vi "Cal Attendance.vi"(8 "error in (no error)":errorcluster, 11 "AttendRecord.lvclass":refnum<class "AttendRecord.lvclass">) -> (0 "error out":errorcluster, 3 "AttendRecord.lvclass":refnum<class "AttendRecord.lvclass">)   [LabVIEW 2015]
uses:
  AttendRecord.lvclass
panel:
  in  "Calendances(\"\")":string[][](array[string])
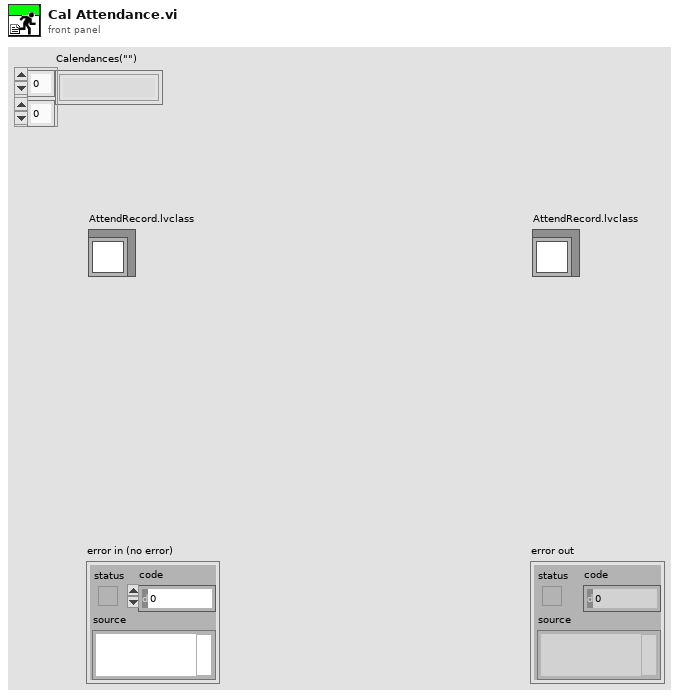
[diagram p1: front panel]
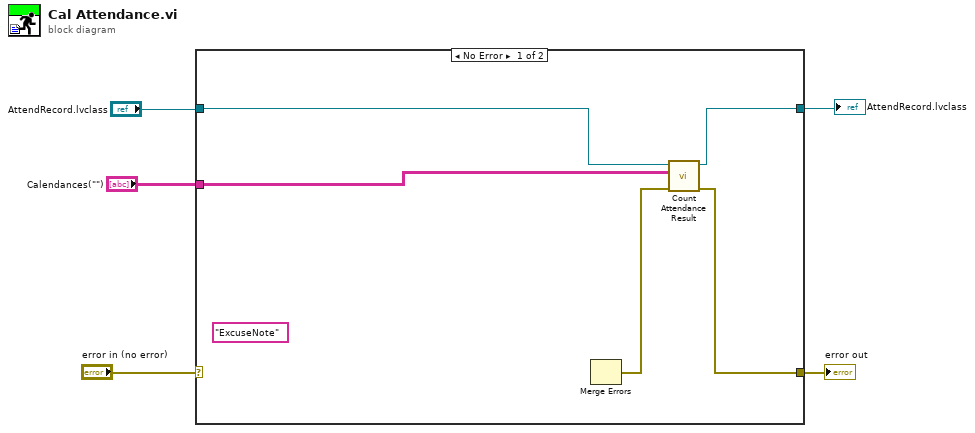
[diagram p0: block diagram]
diagram:
  n1 = case shown="No Error" "error in (no error)" {
    selector: "error in (no error)" -> [_ w12]
    tunnel: [w9 w12] -> w4
    tunnel: [w7 w11] -> w2
    tunnel: "AttendRecord.lvclass" -> [w8 w11]
    tunnel: "Calendances(\"\")" -> [w6 _]
    frame No Error {
      (unwired) "ExcuseNote" ("string")
      n2 = Merge Errors() -> (w10:errorcluster)  [unwired: 3 in]
      n3 = call "Count Attendance Result.vi"("error in (no error)"=w10, "Calendances(\"\")"=w6, "AttendRecord.lvclass"=w8) -> ("error out"=w9:errorcluster, "AttendRecord.lvclass Out"=w7:refnum<class "AttendRecord.lvclass">)  [unwired: 7 in]
    }
    frame Error {
    }
  }
  "error out" <- w4
  "AttendRecord.lvclass" <- w2
